vi "Untitled 2.vi"(8 "error in (no error)":errorcluster, 10 "Boolean":bool) -> (0 "error out":errorcluster)   [LabVIEW 2015]
panel:
  out "Motor Output 2":dbl
  out "Motor Output":dbl
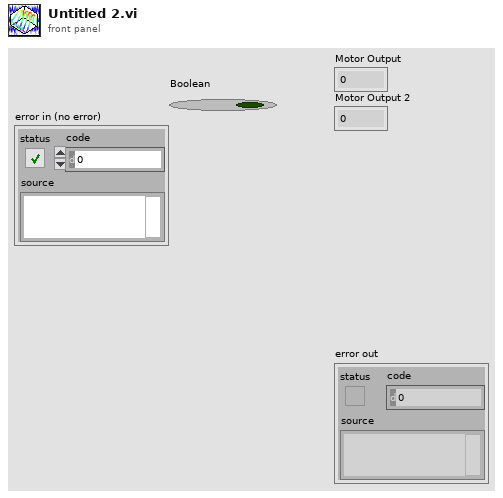
[diagram p1: front panel]
types:
  T1 = typedef "WPI_MotorControlDeviceRef.ctl" = cluster{"DeviceStatus":errorcluster, "Type":T2, "PWM":cluster{"PWM Channel":T3, "DeadBand":T4}, "CAN":cluster{"Device Number":u8, "Control Mode":T5, "Semaphore":T6, "Max Vout":dbl, "TalonSRX Control Mode":T7}, "Invert":bool}
  T2 = typedef "WPI_MotorControlType.ctl" = enum16{"PWM", "CAN", "CANTalonSRX"}
  T3 = typedef "FPGA_DIOPWMChannel.ctl" = enum8{"PWM 0", "PWM 1", "PWM 2", "PWM 3", "PWM 4", "PWM 5", "PWM 6", "PWM 7", "PWM 8", "PWM 9", "PWM MXP 0", "PWM MXP 1", "PWM MXP 2", "PWM MXP 3", "PWM MXP 4", "PWM MXP 5", "PWM MXP 6", "PWM MXP 7", "PWM MXP 8", "PWM MXP 9", "Invalid"}
  T4 = typedef "WPI_PWMDeadband.ctl" = cluster{"Name":string, "maxPositivePwm":i32, "minPositivePwm":i32, "centerPwm":i32, "maxNegativePwm":i32, "minNegativePwm":i32, "angularRange":u16}
  T5 = typedef "WPI_CANJaguar_ControlMode.ctl" = enum8{"Percent VBus", "Current", "Speed", "Position", "Voltage"}
  T6 = typedef "Semaphore RefNum" = refnum<k1>
  T7 = typedef "WPI_CANTalonSRX_APIControlMode.ctl" = enum8{"Percent VBus", "Speed", "Position", "Slave", "Unchanged / Invalid", "Voltage Compensation", "Current", "Motion Profile"}
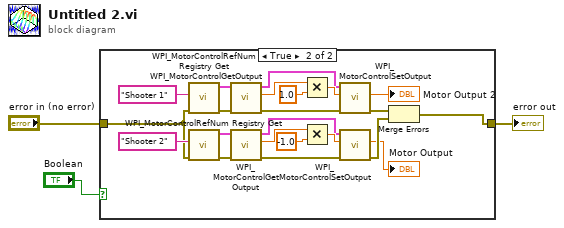
[diagram p0: block diagram]
diagram:
  n1 = case shown="True" "Boolean" {
    tunnel: "error in (no error)" -> [w4 w16]
    tunnel: [w4 w9] -> w2
    frame False {
    }
    frame True {
      n2 = call <vilib>:"WPI_MotorControlRefNum Registry Get.vi"("error in (no error)"=w16, "refnum name"="Shooter 1") -> ("error out"=w20:errorcluster, "MotorControlDevRef"=w19:T1)  [unwired: 8 in]
      n3 = call <vilib>:"WPI_MotorControlRefNum Registry Get.vi"("error in (no error)"=w16, "refnum name"="Shooter 2") -> ("error out"=w24:errorcluster, "MotorControlDevRef"=w22:T1)  [unwired: 8 in]
      n4 = call <vilib>:"WPI_MotorControlGetOutput.vi"("error in (no error)"=w20, "MotorControlDevRef"=w19) -> ("error out"=w10:errorcluster, "Output"=w17:dbl, "MotorControlDevRef"=w11:T1)  [unwired: 7 in]
      n5 = call <vilib>:"WPI_MotorControlGetOutput.vi"("error in (no error)"=w24, "MotorControlDevRef"=w22) -> ("error out"=w13:errorcluster, "Output"=w23:dbl, "MotorControlDevRef"=w12:T1)  [unwired: 7 in]
      n6 = Multiply(x=w17, y=1.0) -> (x*y=w14:dbl)
      n7 = Multiply(x=w23, y=-1.0) -> (x*y=w15:dbl)
      n8 = call <vilib>:"WPI_MotorControlSetOutput.vi"("error in (no error)"=w10, "Output"=w14, "MotorControlDevRef"=w11) -> ("error out"=w8:errorcluster, "Motor Output"=→"Motor Output 2":dbl)  [unwired: 6 in, 1 out]
      n9 = call <vilib>:"WPI_MotorControlSetOutput.vi"("error in (no error)"=w13, "Output"=w15, "MotorControlDevRef"=w12) -> ("error out"=w7:errorcluster, "Motor Output"=→"Motor Output":dbl)  [unwired: 6 in, 1 out]
      n10 = Merge Errors(w8, w7) -> (w9:errorcluster)
    }
  }
  "error out" <- w2
